vi "Read Camera Name.vi"(8 "error in":errorcluster, 10 "IMAQdx Data":T3 {"SerialNumberHigh" format="%x"; "SerialNumberLow" format="%x"}, 11 "Config Manager in":refnum<class "Config Manager Class.lvclass">) -> (0 "error out":errorcluster, 2 "Camera Data":T2, 3 "Config Manager out":refnum<class "Config Manager Class.lvclass">)   [LabVIEW 2011, in "Config Manager Class.lvclass"]
uses:
  Config Manager Class.lvclass
  Type Definitions/Camera Enum.ctl
  Config Manager Class.lvclass/Config Manager Class.ctl
  <vilib>/Utility/config.llb/Read Key (U32).vi
  <vilib>/Utility/config.llb/Read Key (String).vi
  <vilib>/Utility/config.llb/Read Key (Double).vi
  <vilib>/Utility/config.llb/NI_LVConfig.lvlib
panel:
  out "VOID":T1
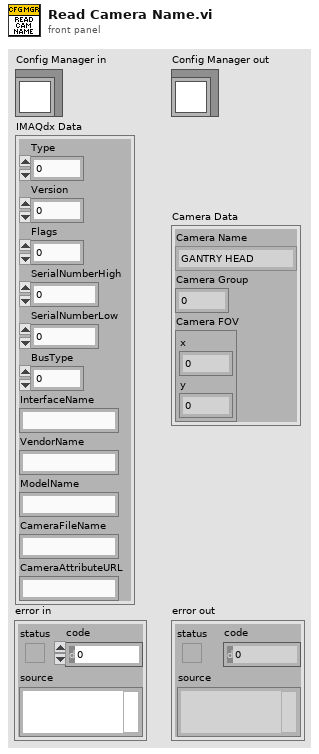
[diagram p1: front panel]
types:
  T1 = typedef "Camera Enum.ctl" = enum16{"GANTRY HEAD", "NEEDLE CALIBRATION X", "NEEDLE CALIBRATION Y"}
  T2 = cluster{"Camera Name":T1, "Camera Group":u32, "Camera FOV":cluster{"x":dbl, "y":dbl}}
  T3 = cluster{"Type":u32, "Version":u32, "Flags":u32, "SerialNumberHigh":u32, "SerialNumberLow":u32, "BusType":u32, "InterfaceName":string, "VendorName":string, "ModelName":string, "CameraFileName":string, "CameraAttributeURL":string}
  T4 = typedef "NI_LVConfig.lvlib/Config Data RefNum.ctl" = refnum<k1>
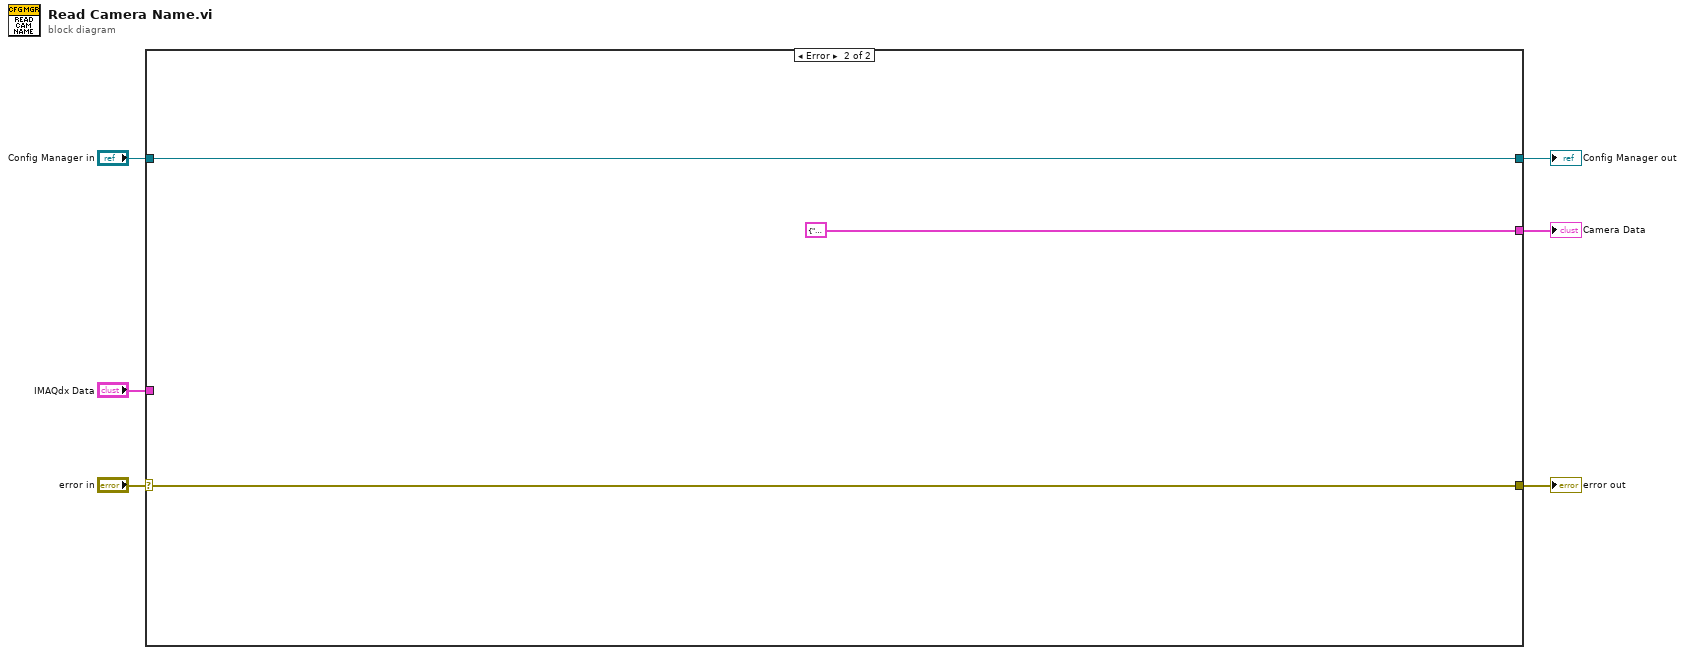
[diagram p0: block diagram]
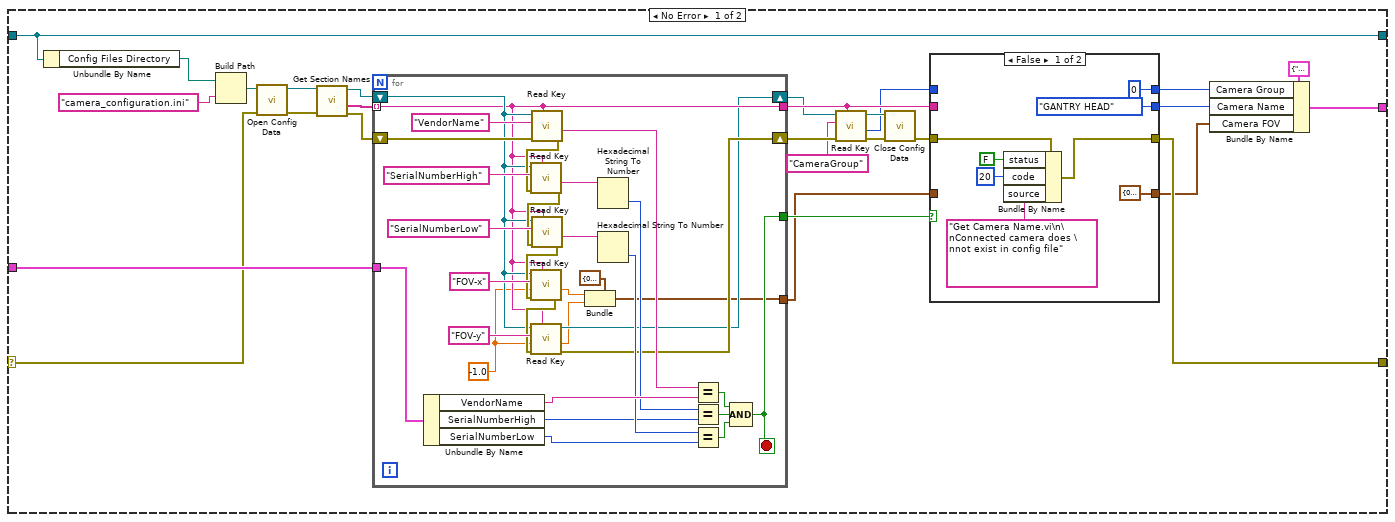
[diagram p2: hidden frame]
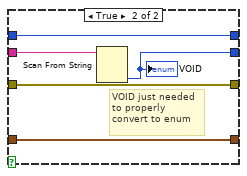
[diagram p3: hidden frame]
diagram:
  n1 = case shown="Error" "error in" {
    selector: "error in" -> [w14 w80]
    tunnel: "IMAQdx Data" -> [w28 _]
    tunnel: "Config Manager in" -> [w13 w81]
    tunnel: [w13 w81] -> w3
    tunnel: [w12 w80] -> w2
    tunnel: [w8 T2 {"Camera Name"=enum."GANTRY HEAD", "Camera Group"=0, "Camera FOV"={"x"=0.0, "y"=0.0}} ("Camera Data 2")] -> w1
    frame No Error {
      n2 = Unbundle By Name(w13) -> ("Config Files Directory"=w15:path)
      n3 = Build Path(base path=w15, name or relative path="camera_configuration.ini") -> (appended path=w32:path)
      n4 = call <vilib>:"Open Config Data.vi"("error in (no error)"=w14, "configuration file path"=w32) -> ("error out"=w31:errorcluster, "refnum"=w30:T4)  [unwired: 7 in, 1 out]
      n5 = call <vilib>:"Get Section Names.vi"("error in (no error)"=w31, "refnum"=w30) -> ("error out"=w26:errorcluster, "section names"=w29:string[], "refnum out"=w27:T4)  [unwired: 7 in]
      n6 = for {
        tunnel: w29 -> [w54] mode=indexing
        tunnel: w28 -> [w74]
        tunnel: [w66] -> w25
        tunnel: [w54] -> w21
        shift-right: [w53] -> w22
        shift-left: w26 -> [w69]
        shift-right: [w52] -> w19
        shift-left: w27 -> [w55]
        tunnel: [w47] -> w16
        stop <- w66 stop-if-true
        w51 = -1.0
        n7 = Unbundle By Name(w74) -> ("VendorName"=w73:string, "SerialNumberHigh"=w60:u32, "SerialNumberLow"=w63:u32)
        n8 = call-poly <vilib>:"Read Key.vi"("section"=w54, "error in (no error)"=w69, "key"="VendorName", "refnum"=w55) -> ("error out"=w68:errorcluster, "value"=w75:string)  [unwired: 4 in, 2 out]
        n9 = call-poly <vilib>:"Read Key.vi"("section"=w54, "error in (no error)"=w68, "key"="SerialNumberHigh", "refnum"=w55) -> ("error out"=w67:errorcluster, "value"=w65:string)  [unwired: 4 in, 2 out]
        n10 = call-poly <vilib>:"Read Key.vi"("section"=w54, "error in (no error)"=w67, "key"="SerialNumberLow", "refnum"=w55) -> ("error out"=w57:errorcluster, "value"=w64:string)  [unwired: 4 in, 2 out]
        n11 = call-poly <vilib>:"Read Key.vi"("section"=w54, "error in (no error)"=w57, "default value"=w51, "key"="FOV-x", "refnum"=w55) -> ("error out"=w56:errorcluster, "value"=w49:dbl)  [unwired: 3 in, 2 out]
        n12 = call-poly <vilib>:"Read Key.vi"("section"=w54, "error in (no error)"=w56, "default value"=w51, "key"="FOV-y", "refnum"=w55) -> ("error out"=w53:errorcluster, "value"=w48:dbl, "refnum out"=w52:T4)  [unwired: 3 in, 1 out]
        n13 = Bundle(cluster=cluster{"x":dbl, "y":dbl} {"x"=0.0, "y"=0.0}, "x"=w49, "y"=w48) -> (w47:cluster{"x":dbl, "y":dbl})
        n14 = Hexadecimal String To Number(string=w65) -> (number=w61:u32)  [unwired: 2 in, 1 out]
        n15 = Hexadecimal String To Number(string=w64) -> (number=w62:u32)  [unwired: 2 in, 1 out]
        n16 = Equal?(x=w75, y=w73) -> (x = y?=w72:bool)
        n17 = Equal?(x=w61, y=w60) -> (x = y?=w71:bool)
        n18 = Equal?(x=w62, y=w63) -> (x = y?=w70:bool)
        n19 = Compound Arithmetic op=AND(w72, w71, w70) -> (w66:bool)
      }
      n20 = call-poly <vilib>:"Read Key.vi"("section"=w21, "error in (no error)"=w22, "key"="CameraGroup", "refnum"=w19) -> ("error out"=w23:errorcluster, "value"=w17:u32, "refnum out"=w20:T4)  [unwired: 4 in, 1 out]
      n21 = call <vilib>:"Close Config Data.vi"("error in (no error)"=w23, "refnum"=w20) -> ("error out"=w24:errorcluster)  [unwired: 8 in, 1 out]
      n22 = case shown="False" w25 {
        tunnel: w21 -> [_ w43]
        tunnel: [w40 w46] -> w12
        tunnel: w24 -> [w41 w46]
        tunnel: w17 -> [_ w45]
        tunnel: [u32 0 ("value") w45] -> w9
        tunnel: [cluster{"x":dbl, "y":dbl} {"x"=0.0, "y"=0.0} w44] -> w10
        tunnel: w16 -> [_ w44]
        tunnel: [Camera_Enum."GANTRY HEAD" ("Camera Name") w42] -> w7
        frame False {
          n23 = Bundle By Name(cluster=w41, "status"=FALSE, "code"=20, "source"="Get Camera Name.vi\n\nConnected camera does \nnot exist in config file") -> (w40:errorcluster)
        }
        frame True {
          # "VOID just needed\nto properly\nconvert to enum"
          n24 = Scan From String(input string=w43) -> (output 1=w42:T1)  [unwired: 4 in, 3 out]
          "VOID" <- w42
        }
      }
      n25 = Bundle By Name(cluster=T2 {"Camera Name"=enum."GANTRY HEAD", "Camera Group"=0, "Camera FOV"={"x"=0.0, "y"=0.0}} ("Camera Data 2"), "Camera Group"=w9, "Camera Name"=w7, "Camera FOV"=w10) -> (w8:T2)
    }
    frame Error {
    }
  }
  "error out" <- w2
  "Config Manager out" <- w3
  "Camera Data" <- w1
